vi "Initialize.vi"(8 "error in":errorcluster, 11 "4-20mA Out Settings In":T1) -> (0 "error out":errorcluster, 1 "Initialized":bool, 3 "4-20mA Out Settings Out":T1)   [LabVIEW 2018, in "Pressure Regulator Library.lvlib"]
uses:
  Pressure Regulator Library.lvlib
  Pressure Regulator Device Settings.ctl
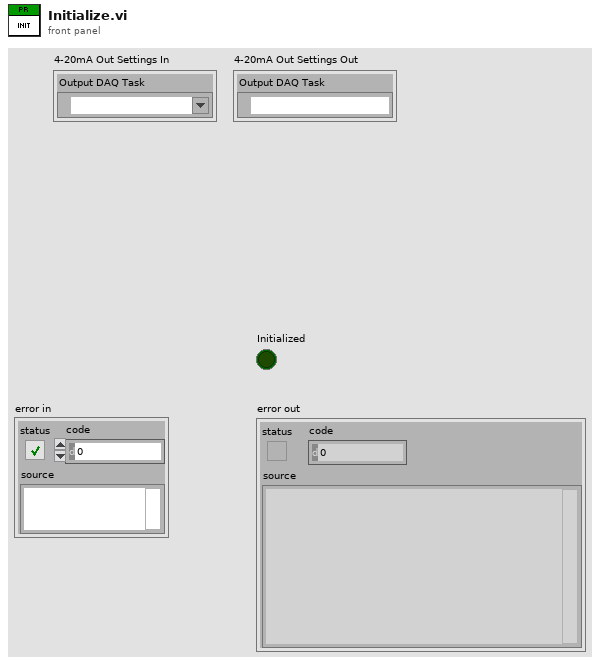
[diagram p1: front panel]
types:
  T1 = typedef "Pressure Regulator Library.lvlib/Pressure Regulator Device Settings.ctl" = cluster{"Output DAQ Task":refnum<k21>}
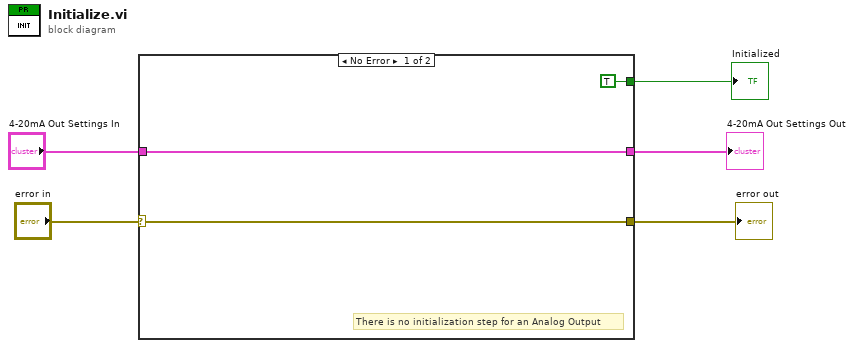
[diagram p0: block diagram]
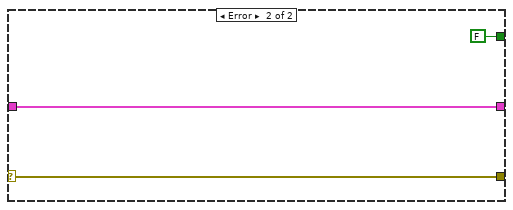
[diagram p2: hidden frame]
diagram:
  n1 = case shown="No Error" "error in" {
    selector: "error in" -> [w8 w10]
    tunnel: [w8 w10] -> w4
    tunnel: "4-20mA Out Settings In" -> [w6 w11]
    tunnel: [w6 w11] -> w1
    tunnel: [TRUE ("Initialized") FALSE ("Initialized")] -> w3
    frame No Error {
      # "There is no initialization step for an Analog Output"
    }
    frame Error {
    }
  }
  "error out" <- w4
  "Initialized" <- w3
  "4-20mA Out Settings Out" <- w1
